vi "Write Pin Map Context.vi"(8 "error in (no error)":errorcluster, 10 "pin map context":T1, 11 "MeasurementContext in":refnum<class "MeasurementContext.lvclass">) -> (0 "error out":errorcluster, 3 "MeasurementContext out":refnum<class "MeasurementContext.lvclass">)   [LabVIEW 2020, in "MeasurementContext.lvclass"]
uses:
  MeasurementContext.lvclass
  RPC Messages/ni_measurements_PinMapContext.ctl
  MeasurementContext.lvclass/MeasurementContext.ctl
  MeasurementTemplate_server.lvlib
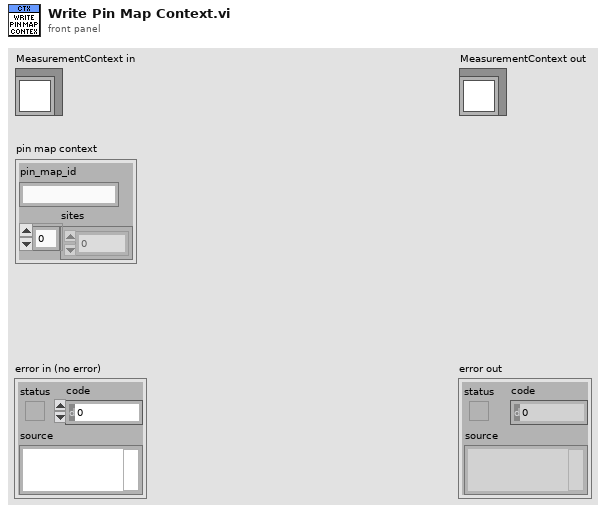
[diagram p1: front panel]
types:
  T1 = typedef "MeasurementTemplate_server.lvlib/ni_measurements_PinMapContext.ctl" = cluster{"pin_map_id":string, "sites":i32[]}
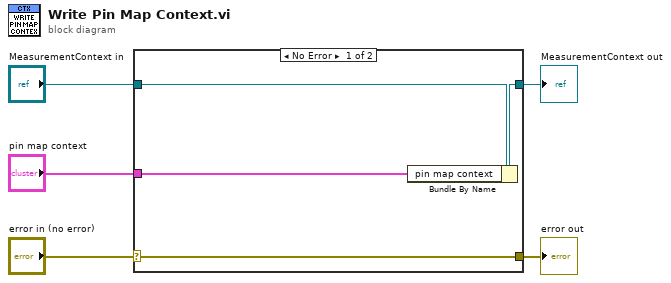
[diagram p0: block diagram]
diagram:
  n1 = case shown="No Error" "error in (no error)" {
    selector: "error in (no error)" -> [w9 w10]
    tunnel: [w9 w10] -> w4
    tunnel: [w7 w11] -> w2
    tunnel: "MeasurementContext in" -> [w8 w11]
    tunnel: "pin map context" -> [w6 _]
    frame No Error {
      n2 = Bundle By Name(cluster=w8, "pin map context"=w6) -> (w7:refnum<class "MeasurementContext.lvclass">)
    }
    frame Error {
    }
  }
  "error out" <- w4
  "MeasurementContext out" <- w2
